vi "控件移位.vi"(8 "错误输入（无错误）":errorcluster, 9 "终点":T1, 10 "起始点":T1 caption="原点", 11 "控件引用输入":refnum<vi>) -> (0 "错误输出":errorcluster, 3 "引用输出":refnum<vi>)   [LabVIEW 8.6, in "窗口操作.lvlib"]
uses:
  <vilib>/Utility/miscctls.llb/LVPositionTypeDef.ctl
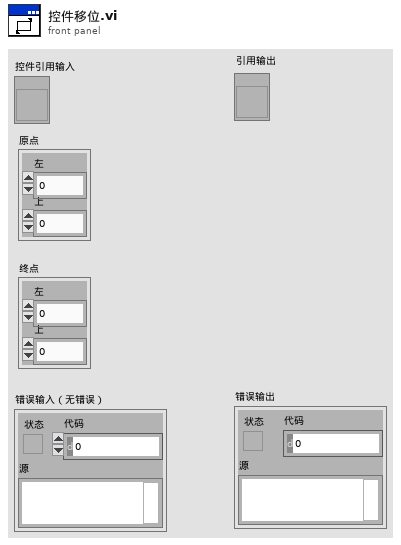
[diagram p1: front panel]
types:
  T1 = typedef "LVPositionTypeDef.ctl" = cluster{"Left":i32, "Top":i32}
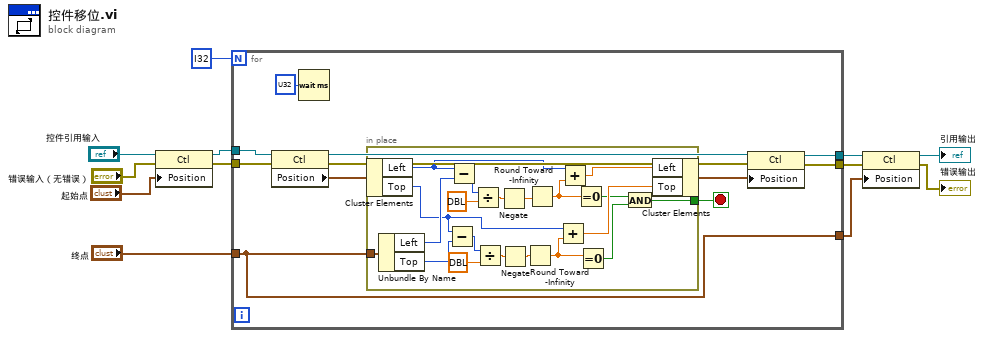
[diagram p0: block diagram]
diagram:
  n1 = property on="Property Node" class="Ctl"(reference="控件引用输入", error in="错误输入（无错误）", "Position"="起始点") -> (reference out=w8:refnum<vi>, error out=w7:errorcluster)
  n2 = for {
    N: i32 ? -> [_]
    tunnel: w8 -> [w21]
    tunnel: [w18] -> w11
    tunnel: "终点" -> [w13]
    tunnel: [w13] -> w10
    tunnel: [w15] -> w9
    tunnel: w7 -> [w14]
    stop <- w19 stop-if-true
    n3 = property on="Property Node" class="Ctl"(reference=w21, error in=w14) -> (reference out=w17:refnum<vi>, error out=w20:errorcluster, "Position"=w23:T1)
    n4 = Wait (ms)(milliseconds to wait=u32 ?) -> ()  [unwired: 1 out]
    n5 = in-place {
      in-place-border: [w33] -> w19
      in-place-border: w13 -> [w32]
      n6 = in-place-cluster #1(w23) -> ("Left"=w41:i32, "Top"=w29:i32)
      n7 = Unbundle By Name(w32) -> ("Left"=w31:i32, "Top"=w30:i32)
      n8 = Subtract(x=w29, y=w30) -> (x-y=w39:i32)
      n9 = Subtract(x=w41, y=w31) -> (x-y=w43:i32)
      n10 = Divide(x=w43, y=dbl ?) -> (x/y=w27:dbl)
      n11 = Divide(x=w39, y=dbl ?) -> (x/y=w26:dbl)
      n12 = Negate(x=w27) -> (-x=w25:dbl)
      n13 = Negate(x=w26) -> (-x=w24:dbl)
      n14 = Round Toward -Infinity(1:w24) -> (0:w40:dbl)
      n15 = Round Toward -Infinity(1:w25) -> (0:w42:dbl)
      n16 = Add(x=w29, y=w40) -> (x+y=w36:dbl)
      n17 = Add(x=w41, y=w42) -> (x+y=w28:dbl)
      n18 = Equal To 0?(x=w42) -> (x = 0?=w34:bool)
      n19 = Equal To 0?(x=w40) -> (x = 0?=w35:bool)
      n20 = And(x=w34, y=w35) -> (x .and. y?=w33:bool)
      n21 = in-place-cluster #1("Left"=w28, "Top"=w36) -> (w16:T1)
    }
    n22 = property on="Property Node" class="Ctl"(reference=w17, error in=w20, "Position"=w16) -> (reference out=w18:refnum<vi>, error out=w15:errorcluster)
  }
  n23 = property on="Property Node" class="Ctl"(reference=w11, error in=w9, "Position"=w10) -> (reference out=→"引用输出":refnum<vi>, error out=→"错误输出":errorcluster)
